vi "channelSort.vi"(8 "triggerMultiplier":i32=500, 9 "InputArray":dbl[][](array[numeric]), 10 "displayRange":i32, 11 "Channels to read":i32) -> (1 "Ch3":dbl[](array[numeric]), 2 "Ch2":dbl[](array[numeric]), 3 "Ch1":dbl[](array[numeric]), 4 "Ch4":dbl[](array[numeric]), 5 "Array":dbl[][](array[numeric]), 6 "VolTrig":dbl[][](array[numeric]))   [LabVIEW 2021]
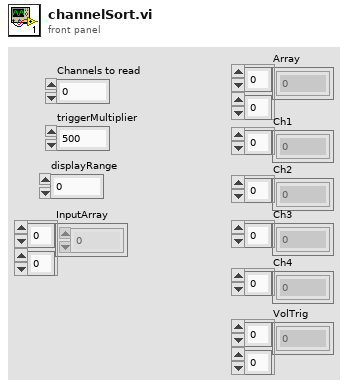
[diagram p1: front panel]
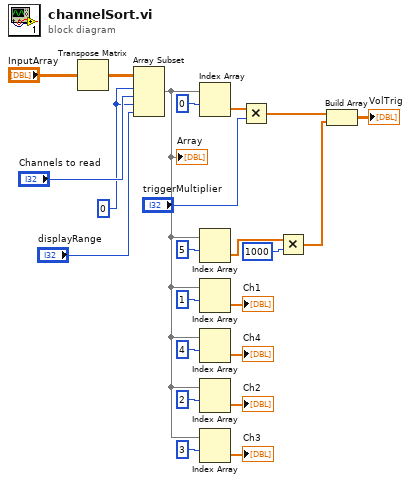
[diagram p0: block diagram]
diagram:
  w7 = 0 ("index")
  n1 = Transpose Matrix(1:"InputArray") -> (0:w17:dbl[][])
  n2 = Array Subset(array=w17, index (row)=w7, length (row)="Channels to read", index (col)=w7, length (col)="displayRange") -> (w23:dbl[][])
  "Array" <- w23
  n3 = Index Array(array=w23, index (row)=0) -> (element=w5:dbl[])  [unwired: 1 in]
  n4 = Index Array(array=w23, index (row)=5) -> (element=w3:dbl[])  [unwired: 1 in]
  n5 = Index Array(array=w23, index (row)=1) -> (element=→"Ch1":dbl[])  [unwired: 1 in]
  n6 = Index Array(array=w23, index (row)=4) -> (element=→"Ch4":dbl[])  [unwired: 1 in]
  n7 = Index Array(array=w23, index (row)=2) -> (element=→"Ch2":dbl[])  [unwired: 1 in]
  n8 = Index Array(array=w23, index (row)=3) -> (element=→"Ch3":dbl[])  [unwired: 1 in]
  n9 = Multiply(x=w5, y="triggerMultiplier") -> (x*y=w4:dbl[])
  n10 = Multiply(x=w3, y=1000 ("index")) -> (x*y=w1:dbl[])
  n11 = Build Array(w4, w1) -> (→"VolTrig":dbl[][])
